vi "m1m3_getEvent_InterlockWarning.vi"(8 "error in (no error)":errorcluster, 11 "logevent_InterlockWarning_Ctl":T1) -> (0 "error out":errorcluster, 2 "function return":i32, 3 "logevent_InterlockWarning_Ctl out":T1)   [LabVIEW 2016, in "SALLV_m1m3.lvlib"]
doc: "int m1m3_shm_getEvent_InterlockWarningLV(m1m3_logevent_InterlockWarningLV *logevent_InterlockWarning_Ctl );"
uses:
  SALLV_m1m3.lvlib
  DataTypes/logevent_InterlockWarning.ctl
  SALLV_m1m3.so
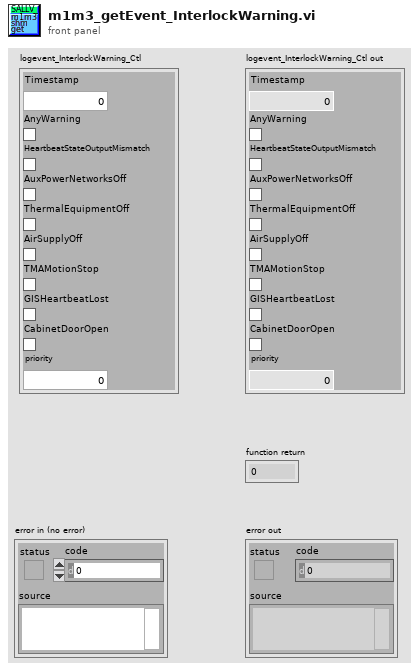
[diagram p1: front panel]
types:
  T1 = typedef "SALLV_m1m3.lvlib/logevent_InterlockWarning.ctl" = cluster{"Timestamp":dbl, "AnyWarning":bool, "HeartbeatStateOutputMismatch":bool, "AuxPowerNetworksOff":bool, "ThermalEquipmentOff":bool, "AirSupplyOff":bool, "TMAMotionStop":bool, "GISHeartbeatLost":bool, "CabinetDoorOpen":bool, "priority":i32}
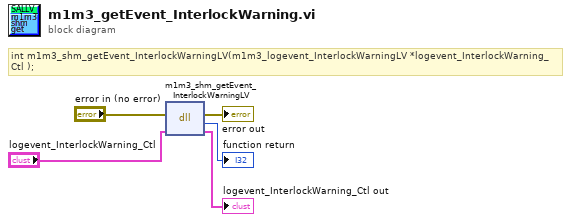
[diagram p0: block diagram]
diagram:
  # "int m1m3_shm_getEvent_InterlockWarningLV(m1m3_logevent_InterlockWarningLV *logevent_InterlockWarning_Ctl );"
  n1 = dll-call lib="opt/CODE/SALLV_m1m3/SALLV_m1m3.*" fn="m1m3_shm_getEvent_InterlockWarningLV"(error in="error in (no error)", "logevent_InterlockWarning_Ctl"="logevent_InterlockWarning_Ctl") -> (error out=→"error out":errorcluster, →"function return":i32, "logevent_InterlockWarning_Ctl"=→"logevent_InterlockWarning_Ctl out":T1)  [unwired: 2 in, 1 out]
